vi "WriteEvtSignal.vi"(8 "error in (no error)":errorcluster, 10 "EvtSignal":variant, 11 "C37.118 Sim in":refnum<class "C37.118 Sim.lvclass">) -> (0 "error out":errorcluster, 3 "C37.118 Sim out":refnum<class "C37.118 Sim.lvclass">)   [LabVIEW 2018, in "SensorPlugins.lvlib" / "C37.118 Sim.lvclass"]
uses:
  C37.118 Sim.lvclass
  C37.118 Sim.lvclass/C37.118 Sim.ctl
  Accessors/Write EvtSignal.vi
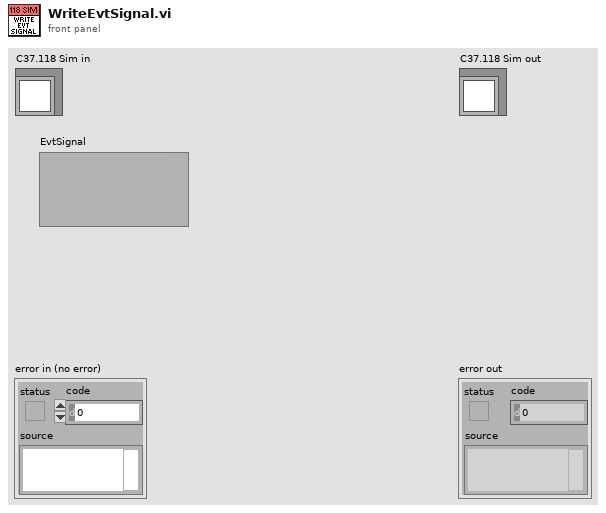
[diagram p1: front panel]
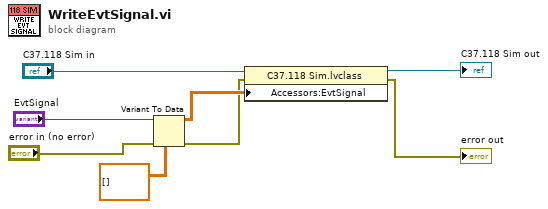
[diagram p0: block diagram]
diagram:
  n1 = Variant To Data(error in="error in (no error)", type=dbl[][] [], Variant="EvtSignal") -> (data=w3:dbl[][], error out=w2:errorcluster)
  n2 = property class="C37.118 Sim.lvclass"(reference="C37.118 Sim in", error in=w2, "Accessors:EvtSignal"=w3) -> (reference out=→"C37.118 Sim out":refnum<class "C37.118 Sim.lvclass">, error out=→"error out":errorcluster)
